vi "voltage_transfer_function.vi"(1 "V_in":fxp<+/-,24,5>) -> (0 "V":fxp<+/-,32,16>)   [LabVIEW 2018]
uses:
  <vilib>/rvi/FXPMathLib/FxpMul/XNode/nifxpmath_Multiplier.xnode
  <vilib>/rvi/FXPMathLib/sim/FxpSim.dll
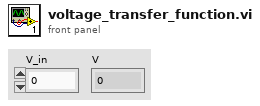
[diagram p1: front panel]
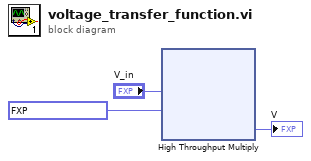
[diagram p0: block diagram]
diagram:
  n1 = xnode "High Throughput Multiply"("x"="V_in", "y"=fxp<+,16,2> 2.79998779296875) -> ("x*y"=→"V":fxp<+/-,32,16>)
